vi "Autonomous Independent.vi"() -> ()   [LabVIEW 2017]
doc: "This VI is called when autonomous begins, and will automatically be terminated when autonomous ends. You can carry out timed or sensor driven robot movement independently without needing to return to the caller."
uses:
  <vilib>/Rock Robotics/Network Tables/NT Read String.vi
  <vilib>/Rock Robotics/Network Tables/NT Write String.vi
panel:
  in  "Robot_Location":bool
  # "Horas para o autonomo:\n\n- Auto 1 - 2 horas, tempo de validação\n\n- Auto 2 - 3 horas de teste\n\n- Auto 3 - 3 horas de teste\n\n- Auto 4 - 5 horas de teste\n\nTotal > 13 horas"
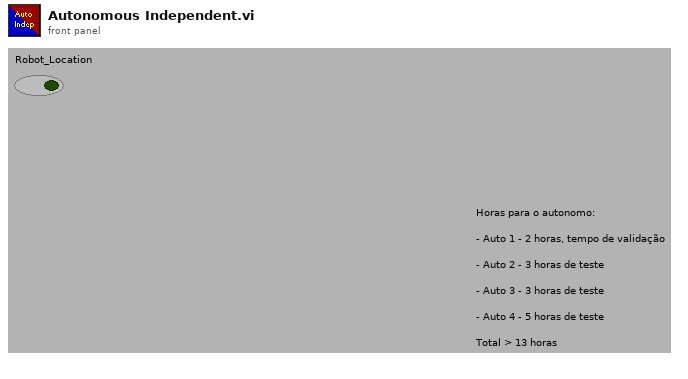
[diagram p1: front panel]
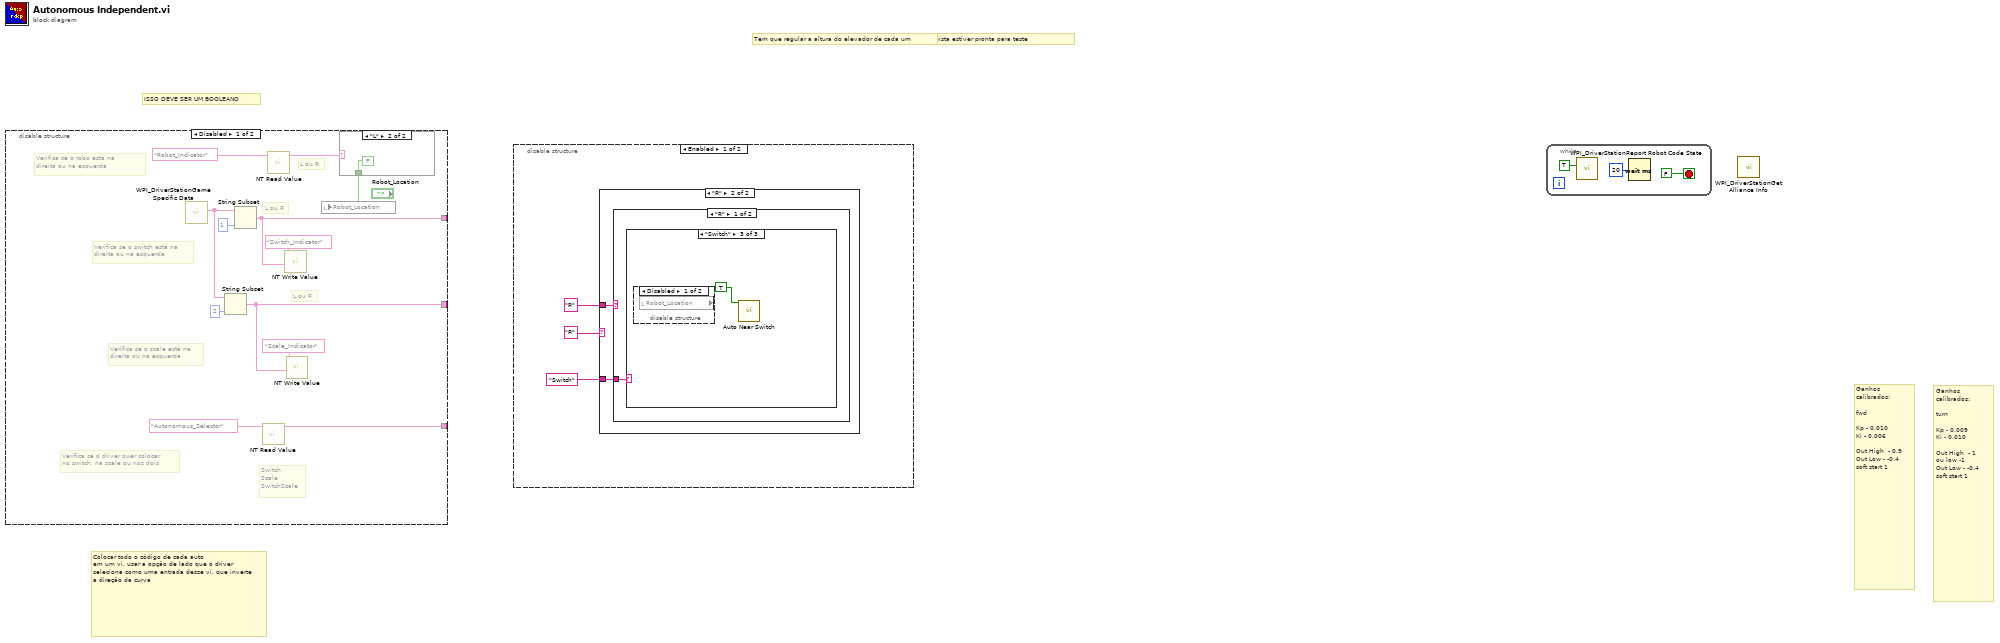
[diagram p0: block diagram]
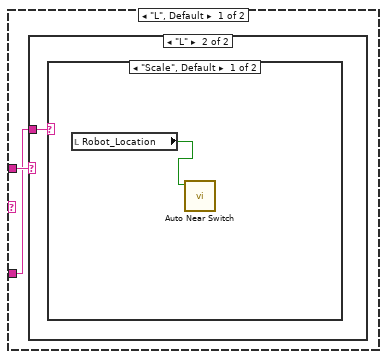
[diagram p2: hidden frame]
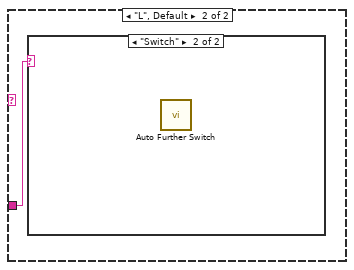
[diagram p9: hidden frame]
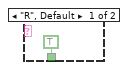
[diagram p12: hidden frame]
diagram:
  # "ISSO DEVE SER UM BOOLEANO"
  # "Colocar todo o código de cada auto\nem um vi, usar a opção de lado que o driver seleciona como uma entrada desse vi, que inverte a direção da curva"
  # "Tem que regular a altura do elevador de cada um"
  # "Tem que regular a distancia de cada quadrado quando a pista estiver pronta para teste"
  # "Ganhos calibrados:\n\nturn\n\nKp - 0.009\nKi - 0.010\n\nOut High  - 1\nou low -1\nOut Low - -0.4\nsoft start 1"
  # "Ganhos calibrados:\n\nfwd\n\nKp - 0.010\nKi - 0.006\n\nOut High  - 0.9\nOut Low - -0.4\nsoft start 1"
  n1 = disable-structure shown="Disabled" {
    disable-tunnel: [w4 _] -> _
    disable-tunnel: [w2 _] -> _
    disable-tunnel: [w6 _] -> _
    frame Disabled {
      # "Verifica se o switch está na\ndireita ou na esquerda"
      # "Switch\nScale\nSwitchScale"
      # "L ou R"
      # "L ou R"
      # "L ou R"
      # "Verifica se o driver quer colocar\nno switch, na scale ou nos dois"
      # "Verifica se o scale está na\ndireita ou na esquerda"
      # "Verifica se o robo está na\ndireita ou na esquerda"
      n2 = call <vilib>:"WPI_DriverStationGame Specific Data.vi"() -> ("Game Specific Data"=w8:string)  [unwired: 11 in]
      n3 = String Subset(string=w8, length (rest)=2 ("length (rest)")) -> (substring=w2:string)  [unwired: 1 in]
      n4 = String Subset(string=w8, length (rest)=1 ("length (rest)")) -> (substring=w4:string)  [unwired: 1 in]
      n5 = call-poly <vilib>:"NT Read Value.vi"("Name"="Autonomous_Selector") -> ("String"=w6:string)  [unwired: 9 in, 1 out]
      n6 = call-poly <vilib>:"NT Read Value.vi"("Name"="Robot_Indicator") -> ("String"=w11:string)  [unwired: 9 in, 1 out]
      n7 = call-poly <vilib>:"NT Write Value.vi"("String"=w4, "Name"="Switch_Indicator") -> ()  [unwired: 9 in, 1 out]
      n8 = call-poly <vilib>:"NT Write Value.vi"("String"=w2, "Name"="Scale_Indicator") -> ()  [unwired: 9 in, 1 out]
      n9 = case shown="\"L\"" w11 {
        tunnel: [TRUE FALSE] -> w1
        frame "R", Default {
        }
        frame "L" {
        }
      }
      n10 = local write "Robot_Location"(w1) -> ()
    }
    frame Enabled {
    }
  }
  n11 = disable-structure shown="Enabled" {
    frame Enabled {
      n12 = case shown="\"R\"" "R" {
        tunnel: "R" -> [w19 w24]
        tunnel: "Switch" -> [w18 w23]
        frame "L", Default {
          n13 = case shown="\"L\"" w19 {
            tunnel: w18 -> [w20 w21]
            frame "R", Default {
              n14 = case shown="\"Switch\", Default" w20 {
                frame "Switch", Default {
                }
                frame "Scale" {
                }
              }
            }
            frame "L" {
              n15 = case shown="\"Scale\", Default" w21 {
                frame "Scale", Default {
                  n16 = local read "Robot_Location"() -> (w22:bool)
                  n17 = call "Auto Near Switch.vi"("Right?"=w22) -> ()  [unwired: 10 in]
                }
                frame "Switch" {
                }
              }
            }
          }
        }
        frame "R" {
          n18 = case shown="\"R\"" w24 {
            tunnel: w23 -> [w25 w27]
            frame "R" {
              n19 = case shown="\"Switch\"" w25 {
                frame "Scale", Default {
                }
                frame "SwitchScale" {
                }
                frame "Switch" {
                  n20 = disable-structure shown="Disabled" {
                    frame Disabled {
                      n21 = local read "Robot_Location"() -> ()  [unwired: 1 out]
                    }
                    frame Enabled {
                    }
                  }
                  n22 = call "Auto Near Switch.vi"("Right?"=TRUE) -> ()  [unwired: 10 in]
                }
              }
            }
            frame "L", Default {
              n23 = case shown="\"Switch\"" w27 {
                frame "Scale", Default {
                }
                frame "Switch" {
                  n24 = call "Auto Further Switch.vi"() -> ()  [unwired: 12 in]
                }
              }
            }
          }
        }
      }
    }
    frame Disabled {
    }
  }
  n25 = while {
    stop <- FALSE stop-if-true
    n26 = call <vilib>:"WPI_DriverStationReport Robot Code State.vi"("Autonomous"=TRUE) -> ()  [unwired: 10 in, 1 out]
    n27 = Wait (ms)(milliseconds to wait=u32 20) -> ()  [unwired: 1 out]
  }
  n28 = call <vilib>:"WPI_DriverStationGet Alliance Info.vi"() -> ()  [unwired: 12 out]
